vi "_builtins_inline_sub_vi.vi"(8 "error in (no error)":errorcluster, 11 "VI Refnum in":refnum<vi>) -> (0 "error out":errorcluster, 3 "VI Refnum out":refnum<vi>)   [LabVIEW 2019, in "Script.lvlib"]
doc: "Inlines the selected SubVI into the owning block diagram.\n\nCreated by: Ryan Pacini"
uses:
  Script.lvlib
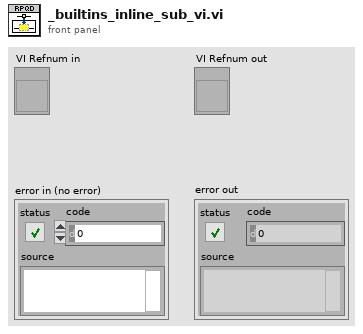
[diagram p1: front panel]
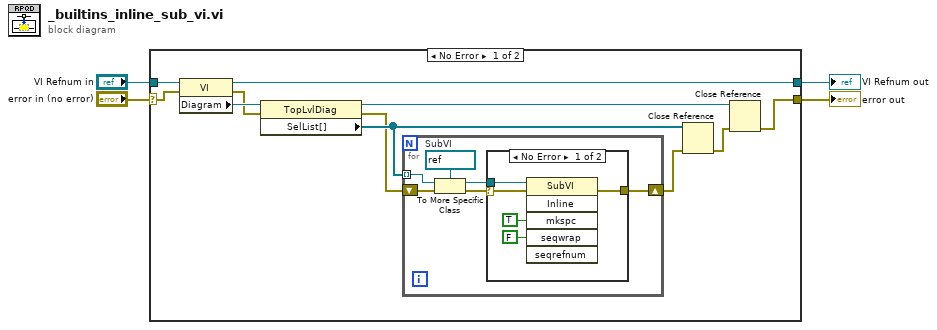
[diagram p0: block diagram]
diagram:
  n1 = case shown="No Error" "error in (no error)" {
    selector: "error in (no error)" -> [w6 w27]
    tunnel: [w15 w28] -> w4
    tunnel: "VI Refnum in" -> [w7 w28]
    tunnel: [w5 w27] -> w1
    frame No Error {
      n2 = property class="VI"(reference=w7, error in=w6) -> (reference out=w15:refnum<vi>, error out=w8:errorcluster, "Diagram"=w13:refnum<vi>)
      n3 = property class="TopLvlDiag"(reference=w13, error in=w8) -> (reference out=w14:refnum<vi>, error out=w9:errorcluster, "SelList[]"=w11:refnum<vi>[])
      n4 = for {
        shift-right: [w19] -> w10
        shift-left: w9 -> [w21]
        tunnel: w11 -> [w16] mode=indexing
        w20 = refnum<vi> refnum  # SubVI
        n5 = To More Specific Class(target class=w20, reference=w16, error in=w21) -> (specific class reference=w18:refnum<vi>, error out=w17:errorcluster)
        n6 = case shown="No Error" w17 {
          selector: w17 -> [w23 _]
          tunnel: [w26 _] -> w19
          tunnel: w18 -> [w24 _]
          frame No Error {
            n7 = invoke class="SubVI" method="Inline"(reference=w24, error in=w23, "mkspc"=TRUE ("Make Space in Block Diagram"), "seqwrap"=FALSE ("Wrap In Sequence? (F)")) -> (error out=w26:errorcluster)  [unwired: 2 in, 5 out]
          }
          frame Error {
          }
        }
      }
      n8 = Close Reference(reference=w11, error in (no error)=w10) -> (error out=w12:errorcluster)
      n9 = Close Reference(reference=w14, error in (no error)=w12) -> (error out=w5:errorcluster)
    }
    frame Error {
    }
  }
  "VI Refnum out" <- w4
  "error out" <- w1
